vi "PRIVATE.ProcCases.vi"(0 "i ref in":refnum<vi>, 1 "selector":string, 2 "Data":T1, 3 "call cluster":T2={"Object"="", "Selector"="", "CallType"=enum."synchronous", "Async Object"="", "Async Selector"="", "Data Descriptor"="", "Data"=[], "Error #"=0, "Expire"=0}, 5 "error in (no error)":errorcluster) -> (14 "i ref out":refnum<vi>, 17 "answer cluster":T2={"Object"="", "Selector"="", "CallType"=enum."synchronous", "Async Object"="", "Async Selector"="", "Data Descriptor"="", "Data"=[], "Error #"=0, "Expire"=0}, 19 "error out":errorcluster)   [LabVIEW 2014, in "NI5112.lvlib"]
doc: "This method is called by a process from within the default case in the event loop. The methods of a class that are linked to events will be called from THIS method. Add your code here."
uses:
  NI5112.lvlib
  CS_Core/CSSystem/CoreLib/CoreLib.lvlib
  CS_Core/BaseProcess/BaseProcess.lvlib
  CS_Core/CSSystem/CoreLib/CoreLib.string 2 byte array.vi
  CS_Core/CSSystem/CoreDefs/CoreDefs.call_type.ctl
  CS_Core/BaseProcess/BaseProcess.descriptor string definition.ctl
  CS_Core/CSSystem/CoreDefs/CoreDefs.rawDataType.ctl
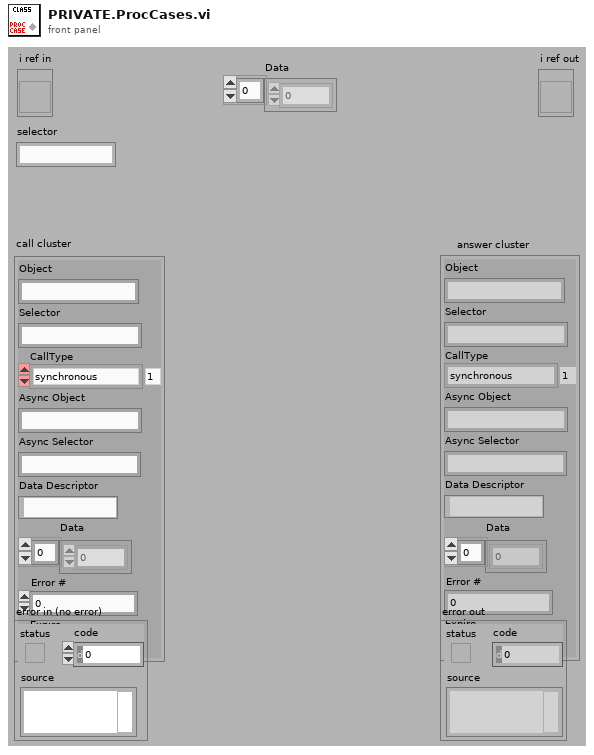
[diagram p1: front panel]
types:
  T1 = typedef "CoreDefs.rawDataType.ctl" = i8[]
  T2 = typedef "CoreDefs.call_type.ctl" = cluster{"Object":string, "Selector":string, "CallType":enum16{"simple", "synchronous", "asynchronous"}, "Async Object":string, "Async Selector":string, "Data Descriptor":T3, "Data":T1, "Error #":i32, "Expire":u32}
  T3 = typedef "BaseProcess.lvlib/BaseProcess.descriptor string definition.ctl" = string
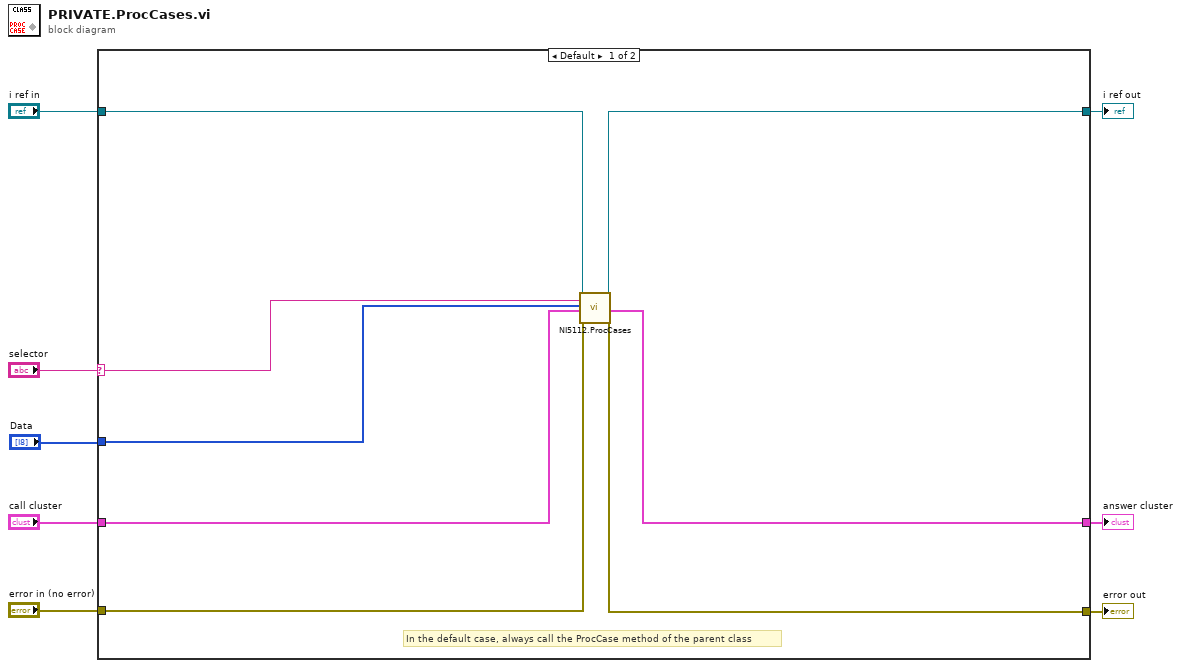
[diagram p0: block diagram]
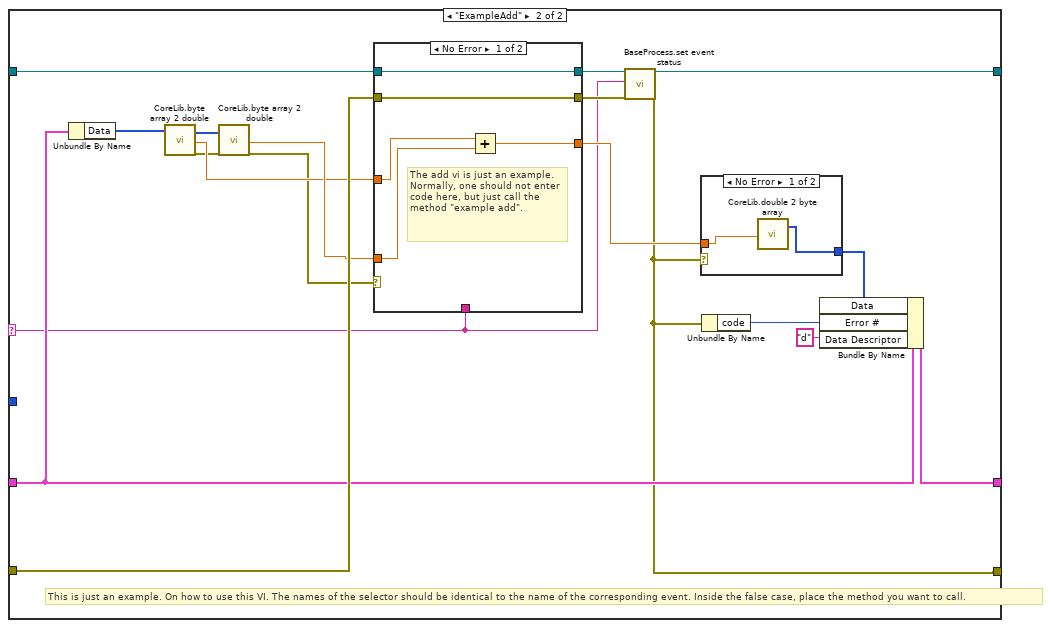
[diagram p2: hidden frame]
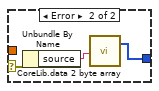
[diagram p3: hidden frame]
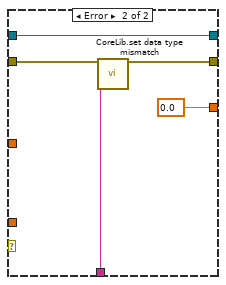
[diagram p4: hidden frame]
diagram:
  n1 = case shown="Default" "selector" {
    selector: "selector" -> [w10 w25]
    tunnel: "Data" -> [w11 _]
    tunnel: "i ref in" -> [w9 w35]
    tunnel: [w16 w24] -> w4
    tunnel: "call cluster" -> [w12 w31]
    tunnel: [w13 w30] -> w7
    tunnel: "error in (no error)" -> [w15 w34]
    tunnel: [w14 w26] -> w2
    frame Default {
      # "In the default case, always call the ProcCase method of the parent class"
      n2 = call "NI5112.ProcCases.vi"("i ref in"=w9, "selector"=w10, "Data"=w11, "call cluster"=w12, "error in (no error)"=w15) -> ("i ref out"=w16:refnum<vi>, "answer cluster"=w13:T2, "error out"=w14:errorcluster)  [unwired: 12 in]
    }
    frame "ExampleAdd" {
      # "This is just an example. On how to use this VI. The names of the selector should be identical to the name of the corresponding event. Inside the false case, place the method you want to call."
      n3 = Unbundle By Name(w31) -> ("Data"=w22:T1)
      n4 = call "CoreLib.byte array 2 double.vi"("byteArray"=w22) -> ("byteArray out"=w21:T1, "d64"=w19:dbl, "error out"=w17:errorcluster)  [unwired: 16 in]
      n5 = call "CoreLib.byte array 2 double.vi"("byteArray"=w21, "error in (no error)"=w17) -> ("d64"=w20:dbl, "error out"=w18:errorcluster)  [unwired: 15 in, 1 out]
      n6 = case shown="No Error" w18 {
        tunnel: [w42 w50] -> w28
        tunnel: w35 -> [w42 w50]
        tunnel: w34 -> [w43 w49]
        tunnel: [w43 w48] -> w27
        tunnel: w20 -> [w45 _]
        tunnel: [w44 0.0] -> w33
        tunnel: w25 -> [_ w46]
        tunnel: w19 -> [w41 _]
        frame No Error {
          # "The add vi is just an example. Normally, one should not enter code here, but just call the method \"example add\"."
          n7 = Add(x=w41, y=w45) -> (x+y=w44:dbl)
        }
        frame Error {
          n8 = call "CoreLib.set data type mismatch.vi"("error in (no error)"=w49, "error source"=w46) -> ("error out"=w48:errorcluster)  [unwired: 17 in]
        }
      }
      n9 = call "BaseProcess.set event status.vi"("i ref in"=w28, "EventStatus"=w25, "error in (no error)"=w27) -> ("i ref out"=w24:refnum<vi>, "error out"=w26:errorcluster)  [unwired: 14 in, 1 out]
      n10 = case shown="No Error" w26 {
        selector: w26 -> [_ w40]
        tunnel: [w36 w39] -> w29
        tunnel: w33 -> [w37 _]
        frame No Error {
          n11 = call "CoreLib.double 2 byte array.vi"("f64"=w37) -> ("byteArray out"=w36:T1)  [unwired: 18 in]
        }
        frame Error {
          n12 = Unbundle By Name(w40) -> ("source"=w38:string)
          n13 = call-poly "CoreLib.data 2 byte array.vi"("string"=w38) -> ("byteArray out"=w39:T1)  [unwired: 18 in]
        }
      }
      n14 = Unbundle By Name(w26) -> ("code"=w32:i32)
      n15 = Bundle By Name(cluster=w31, "Data"=w29, "Error #"=w32, "Data Descriptor"="d") -> (w30:T2)
    }
  }
  "answer cluster" <- w7
  "i ref out" <- w4
  "error out" <- w2
